vi "add EIP tag.vi"(5 "Number of Elements":u32=1, 7 "eip tag types":T1, 8 "error in":errorcluster, 9 "Tag Name":string, 10 "Network Path":string, 11 "EIP Tags configuration in":refnum<class "EIP Tags Configuration.lvclass">) -> (0 "error out":errorcluster, 3 "EIP Tags configuration out":refnum<class "EIP Tags Configuration.lvclass">)   [LabVIEW 2013, in "EIP Tags Configuration.lvclass"]
uses:
  EIP Tags Configuration.lvclass
  eip tag types.ctl
  EIP Tags Configuration.lvclass/EIP Tags Configuration.ctl
  eip tag definition.ctl
  <vilib>/NI/Configuration Framework/NISE_CEF_TreeControl.lvlib
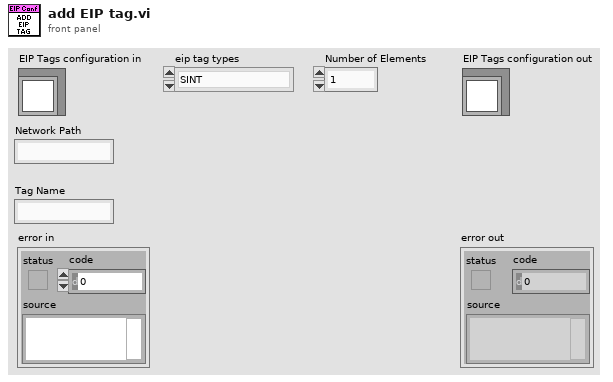
[diagram p1: front panel]
types:
  T1 = typedef "EIP Tags Configuration.lvclass/eip tag types.ctl" = enum16{"SINT", "INT", "DINT", "REAL", "BOOL", "STRING"}
  T2 = typedef "EIP Tags Configuration.lvclass/eip tag definition.ctl" = cluster{"eip tag types":T1, "unique tag name":string, "Number of Elements":u32}
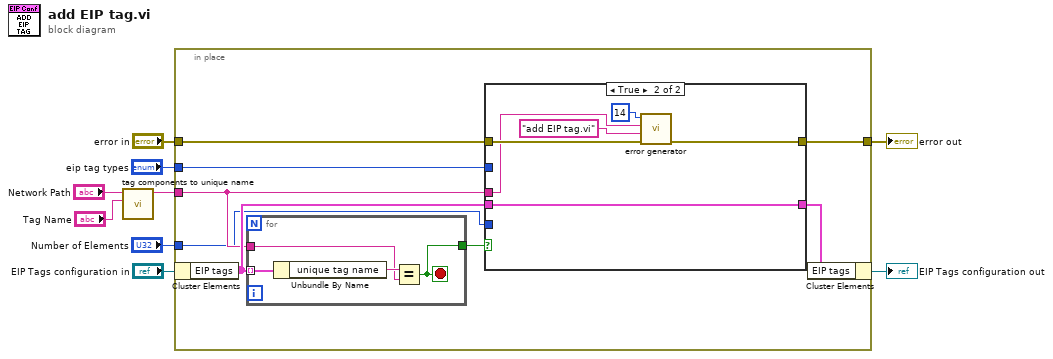
[diagram p0: block diagram]
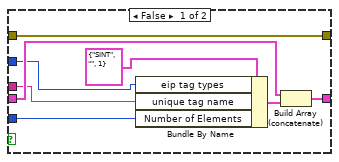
[diagram p2: hidden frame]
diagram:
  n1 = call "tag components to unique name.vi"("Tag Name"="Tag Name", "Network Path"="Network Path") -> ("unique name"=w4:string)  [unwired: 9 in]
  n2 = in-place {
    in-place-border: "error in" -> [w15]
    in-place-border: w4 -> [w12]
    in-place-border: [w16] -> w3
    in-place-border: "eip tag types" -> [w11]
    in-place-border: "Number of Elements" -> [w10]
    n3 = in-place-cluster #1("EIP Tags configuration in") -> ("EIP tags"=w13:T2[])
    n4 = for {
      tunnel: w13 -> [w35] mode=indexing
      tunnel: w12 -> [w33]
      tunnel: [w32] -> w17
      stop <- w32 stop-if-true
      n5 = Unbundle By Name(w35) -> ("unique tag name"=w34:string)
      n6 = Equal?(x=w34, y=w33) -> (x = y?=w32:bool)
    }
    n7 = case shown="True" w17 {
      tunnel: [w21 w31] -> w16
      tunnel: w15 -> [w21 w30]
      tunnel: [w22 w28] -> w14
      tunnel: w13 -> [w24 w28]
      tunnel: w12 -> [w20 w27]
      tunnel: w11 -> [w19 _]
      tunnel: w10 -> [w18 _]
      frame False {
        n8 = Bundle By Name(cluster=T2 {"eip tag types"=enum."SINT", "unique tag name"="", "Number of Elements"=1} ("tag spec"), "eip tag types"=w19, "unique tag name"=w20, "Number of Elements"=w18) -> (w23:T2)
        n9 = Build Array (concatenate)(w24, w23) -> (w22:T2[])
      }
      frame True {
        n10 = call <vilib>:"error generator.vi"("error in"=w30, "source"="add EIP tag.vi", "append error message"=w27, "error code (0)"=14) -> ("error out"=w31:errorcluster)  [unwired: 5 in]
      }
    }
    n11 = in-place-cluster #1("EIP tags"=w14) -> (→"EIP Tags configuration out":refnum<class "EIP Tags Configuration.lvclass">)
  }
  "error out" <- w3
